vi "LaunchGenerator.vi"() -> ()   [LabVIEW 2021]
uses:
  Generator/Generator/Generator.lvclass
  C:/Program Files (x86)/National Instruments/LabVIEW 2021/vi.lib/ActorFramework/Actor/Actor.lvclass
  Generator/Generator Messages/Write NumRange Msg/Write NumRange Msg.lvclass/Write NumRange Msg.ctl
  <vilib>/ActorFramework/Message Enqueuer/Message Enqueuer.lvclass/Message Enqueuer.ctl
  Generator/Generator Messages/Write StringLength Msg/Write StringLength Msg.lvclass/Write StringLength Msg.ctl
  <vilib>/ActorFramework/Reply Msg/Reply Msg.lvclass/Reply Msg.ctl
  7fd6c2e3-5a34-4bbf-a67f-205d0afb060b.vi
  <vilib>/ActorFramework/Message Enqueuer/Enqueue.vi
  <vilib>/ActorFramework/Reply Msg/Send Message And Wait For Response.vi
  Generator/Generator Messages/Write NumRange Msg/Write NumRange Msg.lvclass
  C:/Program Files (x86)/National Instruments/LabVIEW 2021/vi.lib/ActorFramework/Message/Message.lvclass
  Generator/Generator Messages/Write StringLength Msg/Write StringLength Msg.lvclass
  Generator/Generator Messages/GetRandomString Msg/GetRandomString Msg.lvclass
  Generator/Generator Messages/GetRandomNum Msg/GetRandomNum Msg.lvclass
  Generator/Generator Messages/GetDateTimeString Msg/GetDateTimeString Msg.lvclass
  Generator/Generator Messages/Read DateTimeString Msg/Read DateTimeString Msg.lvclass
  C:/Program Files (x86)/National Instruments/LabVIEW 2021/vi.lib/ActorFramework/Reply Msg/Reply Msg.lvclass
  <vilib>/ActorFramework/Reply Msg/Reply Msg.lvclass
  Generator/Generator Messages/Read RandomNum Msg/Read RandomNum Msg.lvclass
  Generator/Generator Messages/Read RandomString Msg/Read RandomString Msg.lvclass
  <vilib>/ActorFramework/Stop Msg/Stop Msg.lvclass
  <vilib>/ActorFramework/Message Priority Queue/Priority Enqueue.vi
  <vilib>/ActorFramework/Actor/Actor.lvclass
panel:
  in  "stop":bool
  out "RandomString":string
  out "RandomNum":dbl
  out "DateTimeString":string
  in  "StringLength":i32
  in  "NumRange":dbl
  # "Launch VI"
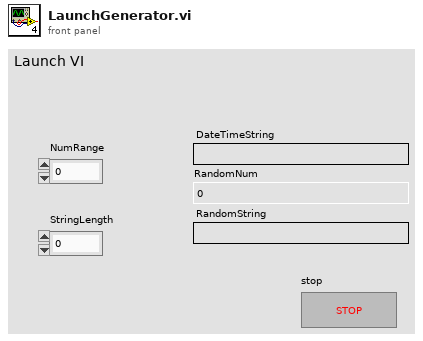
[diagram p1: front panel]
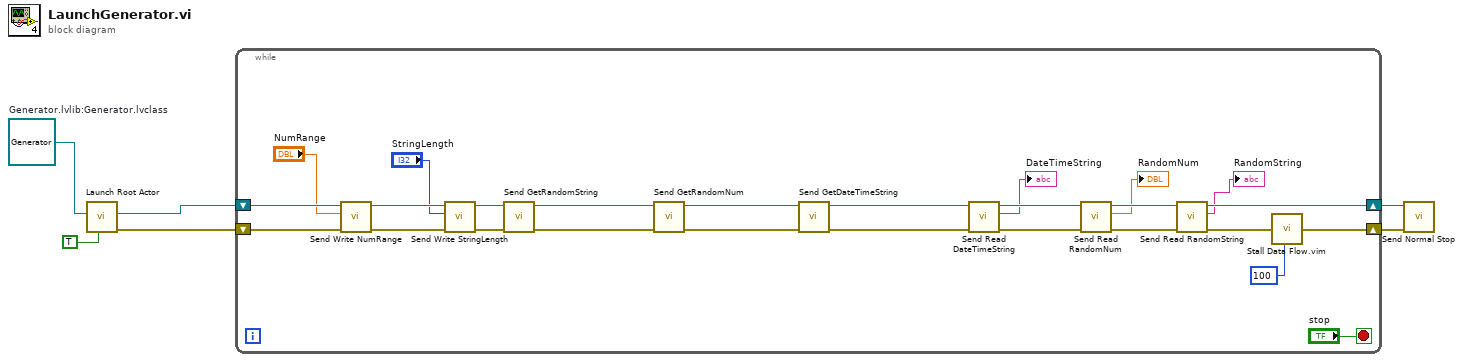
[diagram p0: block diagram]
diagram:
  w6 = refnum<class "Generator.lvclass"> refnum  # Generator.lvlib:Generator.lvclass
  n1 = call <vilib>:"Launch Root Actor.vi"("Open Actor Core front panel? (F)"=TRUE, "Actor"=w6) -> ("error out"=w5:errorcluster, "Actor's Enqueuer"=w3:refnum<class "Message Enqueuer.lvclass">)  [unwired: 8 in]
  n2 = while {
    shift-right: [w9] -> w1
    shift-left: w5 -> [w32]
    shift-right: [w14] -> w2
    shift-left: w3 -> [w26]
    stop <- "stop" stop-if-true
    n3 = call "Send Write NumRange.vi"("error in (no error)"=w32, "NumRange"="NumRange", "Message Enqueuer"=w26) -> ("error out"=w27:errorcluster, "Message Enqueuer out"=w23:refnum<class "Message Enqueuer.lvclass">)  [unwired: 7 in]
    n4 = call "Send Write StringLength.vi"("error in (no error)"=w27, "StringLength"="StringLength", "Message Enqueuer"=w23) -> ("error out"=w24:errorcluster, "Message Enqueuer out"=w22:refnum<class "Message Enqueuer.lvclass">)  [unwired: 7 in]
    n5 = call "Send GetRandomString.vi"("error in (no error)"=w24, "Message Enqueuer"=w22) -> ("error out"=w30:errorcluster, "Message Enqueuer out"=w31:refnum<class "Message Enqueuer.lvclass">)  [unwired: 8 in]
    n6 = call "Send GetRandomNum.vi"("error in (no error)"=w30, "Message Enqueuer"=w31) -> ("error out"=w28:errorcluster, "Message Enqueuer out"=w29:refnum<class "Message Enqueuer.lvclass">)  [unwired: 8 in]
    n7 = call "Send GetDateTimeString.vi"("error in (no error)"=w28, "Message Enqueuer"=w29) -> ("error out"=w19:errorcluster, "Message Enqueuer out"=w20:refnum<class "Message Enqueuer.lvclass">)  [unwired: 8 in]
    n8 = call "Send Read DateTimeString.vi"("error in (no error)"=w19, "Message Enqueuer"=w20) -> ("error out"=w17:errorcluster, "DateTimeString"=→"DateTimeString":string, "Message Enqueuer out"=w18:refnum<class "Message Enqueuer.lvclass">)  [unwired: 7 in]
    n9 = call "Send Read RandomNum.vi"("error in (no error)"=w17, "Message Enqueuer"=w18) -> ("error out"=w15:errorcluster, "RandomNum"=→"RandomNum":dbl, "Message Enqueuer out"=w16:refnum<class "Message Enqueuer.lvclass">)  [unwired: 7 in]
    n10 = call "Send Read RandomString.vi"("error in (no error)"=w15, "Message Enqueuer"=w16) -> ("error out"=w13:errorcluster, "RandomString"=→"RandomString":string, "Message Enqueuer out"=w14:refnum<class "Message Enqueuer.lvclass">)  [unwired: 7 in]
    n11 = call "Stall Data Flow.vim"("value in"=w13, "milliseconds to wait"=u32 100) -> ("value out"=w9:errorcluster)  [unwired: 1 out]
  }
  n12 = call <vilib>:"Send Normal Stop.vi"("error in (no error)"=w1, "Message Enqueuer"=w2) -> ()  [unwired: 9 in, 1 out]
